vi "Read Command _Standby_.vi"(8 "error in (no error)":errorcluster, 11 "SupplyControl in":refnum<class "SupplyControl.lvclass">) -> (0 "error out":errorcluster, 2 "Command \"Standby\"":string, 3 "SupplyControl out":refnum<class "SupplyControl.lvclass">)   [LabVIEW 2019, in "SupplyControl.lvclass"]
uses:
  SupplyControl.lvclass
  SupplyControl.lvclass/SupplyControl.ctl
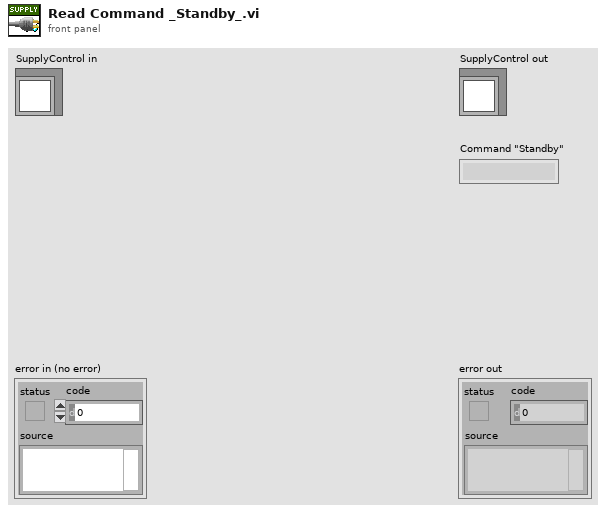
[diagram p1: front panel]
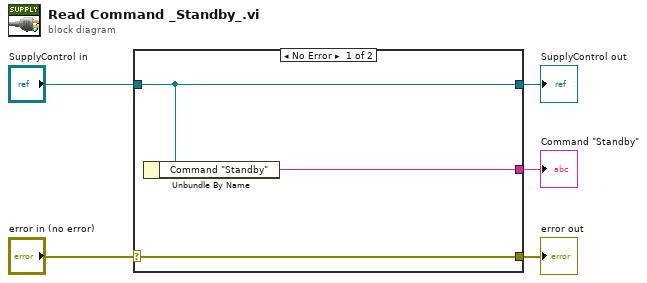
[diagram p0: block diagram]
diagram:
  n1 = case shown="No Error" "error in (no error)" {
    selector: "error in (no error)" -> [w8 w9]
    tunnel: [w8 w9] -> w4
    tunnel: [w7 w10] -> w2
    tunnel: "SupplyControl in" -> [w7 w10]
    tunnel: [w6 _] -> w1
    frame No Error {
      n2 = Unbundle By Name(w7) -> ("Command \"Standby\""=w6:string)
    }
    frame Error {
    }
  }
  "error out" <- w4
  "SupplyControl out" <- w2
  "Command \"Standby\"" <- w1
